vi "CG test stand Loadcell calibration.vi"() -> ()   [LabVIEW 2020]
doc: "This example demonstrates how to read N channels of analog input from a LINX device."
uses:
  <vilib>/MakerHub/LINX/Public/Peripherals/Analog/Analog Read N Chans.vi
  <vilib>/MakerHub/LINX/Private/Local IO/LinxAnalogRead.vi
  <vilib>/MakerHub/LINX/Public/Utilities/Check Channel.vi
  <vilib>/MakerHub/LINX/Public/Utilities/Open Serial.vi
  <vilib>/MakerHub/LINX/Private/Utilties/Generate Error.vi
  <vilib>/Analysis/Matrix/Numeric/Conversions/Array To Matrix - RA.vi
  <vilib>/Utility/file.llb/Write Delimited Spreadsheet (DBL).vi
  <vilib>/MakerHub/LINX/LMH-LINX.lvlib
  <vilib>/Analysis/Matrix/NI_Matrix.lvlib
panel:
  out "Unfiltered":dbl(graph)
  in  "Current Weight":dbl
  out "Filtered Data":dbl
  out "WRITING TO FILE":bool
  in  "?":bool
  out "error out":errorcluster
  out "Full filepath":string
  in  "Path":path
  in  "File extension":string
  in  "Filename":string
  in  "Analog Port":dbl
  out "Time Stamp":timestamp
  out "Filtered":dynamicdata(graph)
  out "Voltage":dbl
  in  "Stop Button":bool
  out "Loop Rate (Hz)":u32
  in  "Serial Port":refnum<visa-resource-name>
  # "X"
  # "+"
  # "CG test stand analog read\n\nThis VI works to read one single voltage value from an Arduino. Currently configured for a Mega 2560."
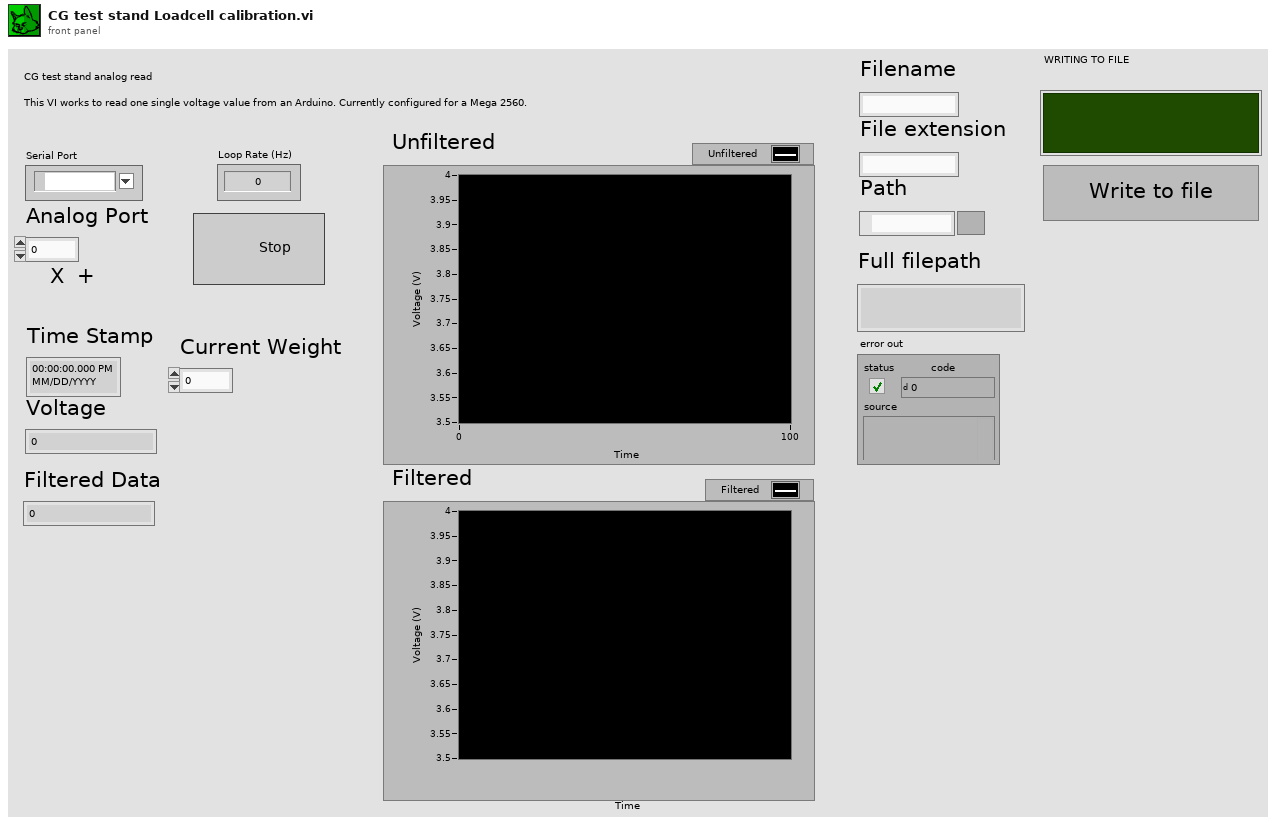
[diagram p1: front panel]
types:
  T1 = typedef "LMH-LINX.lvlib/LINX Ref.ctl" = cluster{"IO":T2, "Interface":T3, "LINX Device Config":T4}
  T2 = typedef "LMH-LINX.lvlib/Platform.ctl" = enum16{"Remote", "Local"}
  T3 = typedef "LMH-LINX.lvlib/Interface.ctl" = enum16{"Serial", "TCP"}
  T4 = typedef "LMH-LINX.lvlib/Device.lvlib/LINX Device Config.ctl" = cluster{"Interface":T3, "COM Port":refnum<visa-resource-name>, "TCP Configuration":T5, "Device Family":u8, "Device ID":u8, "Device Name":string, "TCP Ref":refnum<k5>, "Channels":T6}
  T5 = typedef "LMH-LINX.lvlib/Device.lvlib/TCP Config.ctl" = cluster{"IP Address":string, "Port":u16}
  T6 = typedef "LMH-LINX.lvlib/Channels.ctl" = cluster{"DI":u8[], "DO":u8[], "AI":u8[], "AO":u8[], "PWM":u8[], "QE":u8[], "UART":u8[], "I2C 2":u8[], "SPI":u8[], "CAN":u8[], "Servo":u8[], "AI Ref (V)":dbl, "AI Resolution (Bits)":u8, "AO Ref (V)":dbl, "AO Resolution (Bits)":u8}
  T7 = typedef "NI_Matrix.lvlib/RealMatrix.ctl" = dbl[][]
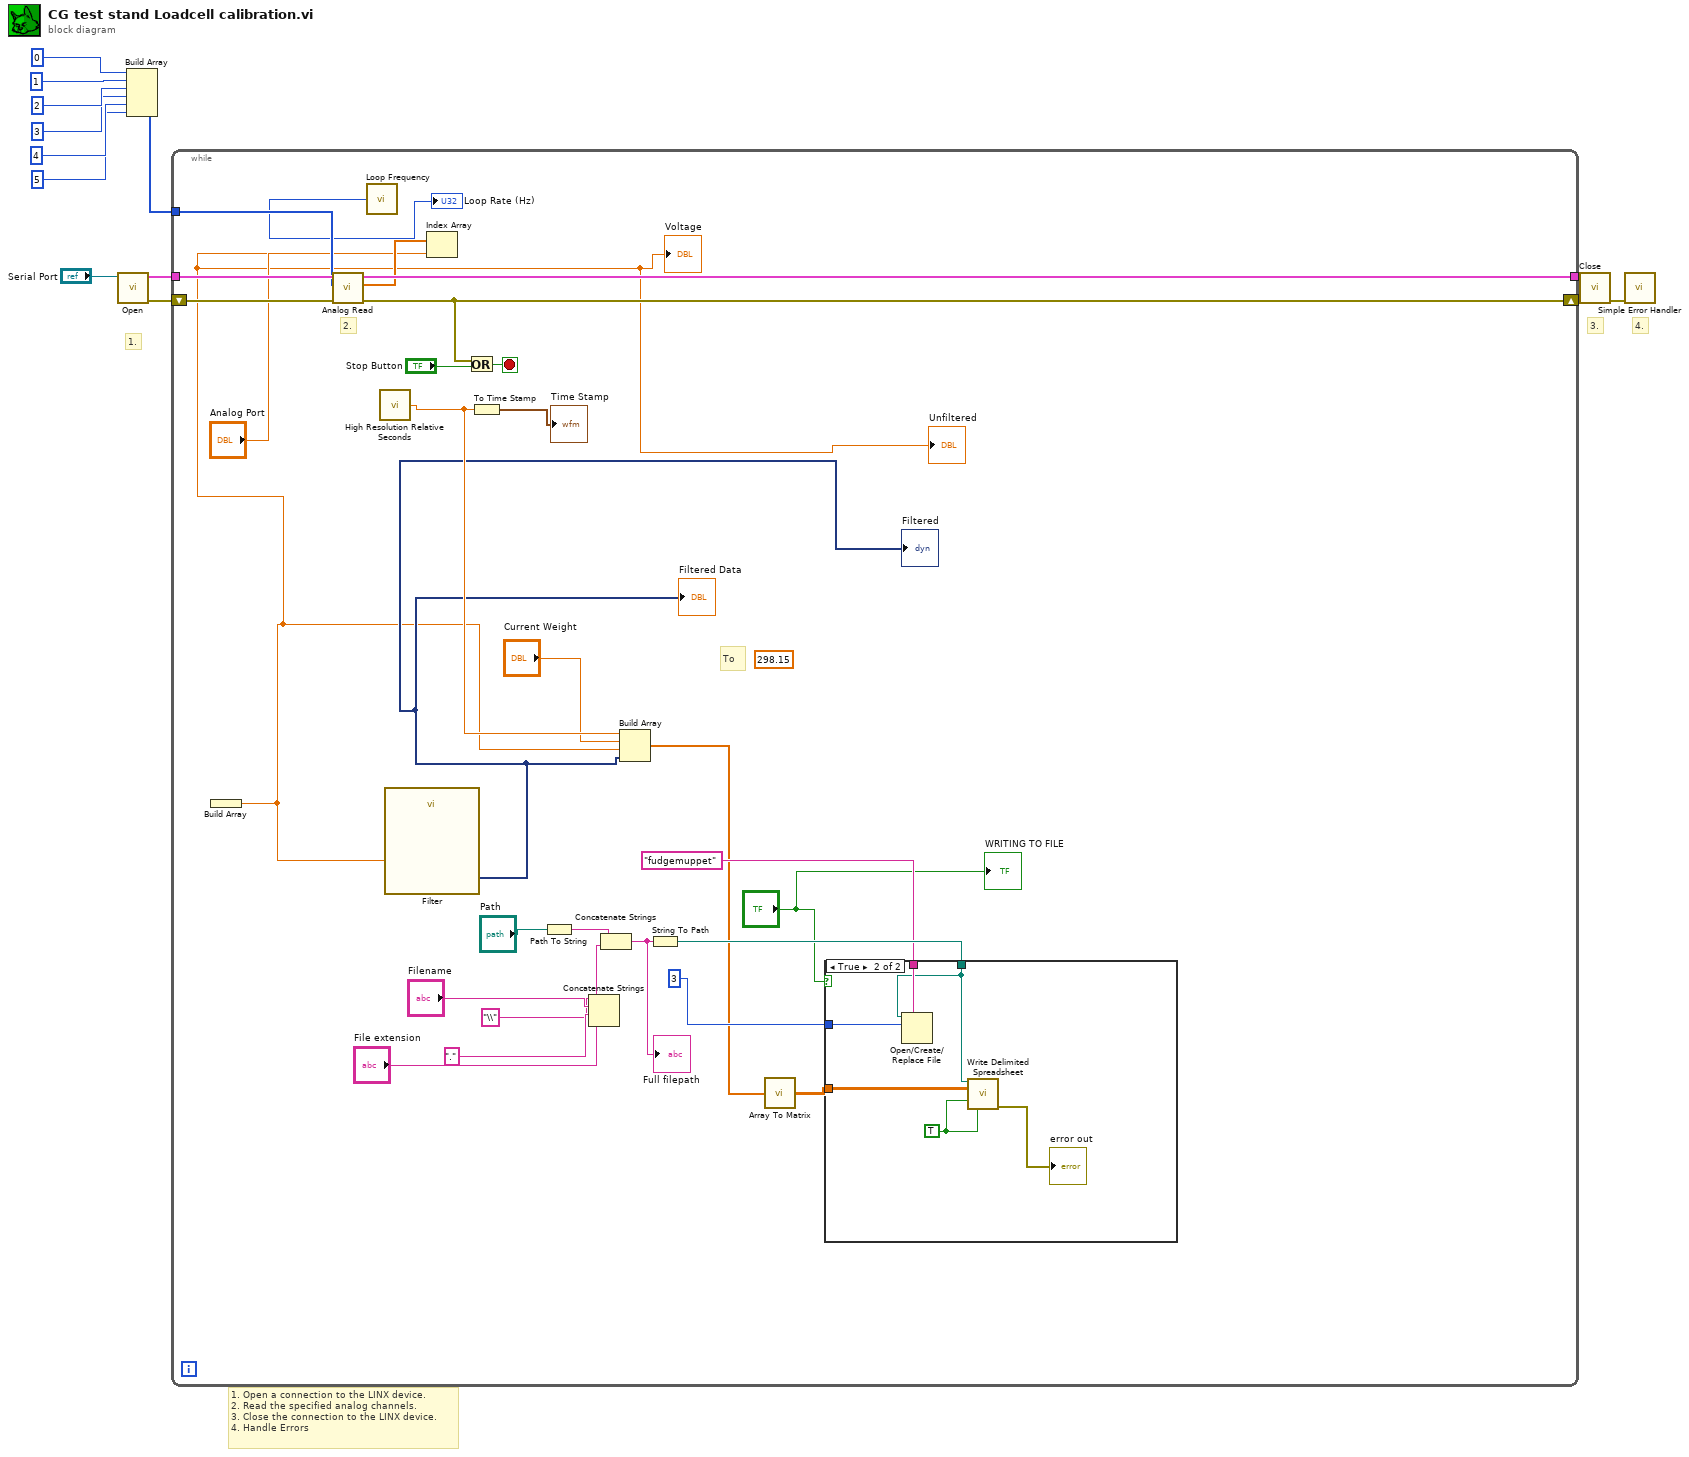
[diagram p0: block diagram]
diagram:
  # "1. Open a connection to the LINX device.\n2. Read the specified analog channels.\n3. Close the connection to the LINX device.\n4. Handle Errors"
  # "4."
  # "3."
  # "1."
  n1 = call-poly <vilib>:"Open.vi"("Serial Port"="Serial Port") -> ("Error Out"=w12:errorcluster, "LINX Resource"=w13:T1)  [unwired: 8 in, 1 out]
  n2 = Build Array(0, 1, 2, 3, 4, 5) -> (w7:i32[])
  n3 = while {
    tunnel: w13 -> [w42]
    tunnel: [w40] -> w11
    shift-right: [w37] -> w10
    shift-left: w12 -> [w41]
    tunnel: w7 -> [w36]
    stop <- w39 stop-if-true
    (unwired) 298.15
    # "To"
    # "2."
    n4 = call-poly <vilib>:"Analog Read.vi"("Error In"=w41, "AI Channel(s)"=w36, "LINX Resource"=w42) -> ("Error Out"=w37:errorcluster, "Voltages"=w35:dbl[], "LINX Resource"=w40:T1)  [unwired: 5 in, 1 out]
    n5 = call <vilib>:"Loop Frequency.vi"() -> ("Loop Rate (Hz)"=→"Loop Rate (Hz)":u32)
    n6 = call <vilib>:"High Resolution Relative Seconds.vi"() -> ("relative seconds"=w18:dbl)
    n7 = Index Array(array=w35, index="Analog Port") -> (element=w14:dbl)
    "Voltage" <- w14
    "Unfiltered" <- w14
    n8 = Build Array(w14) -> ()  [unwired: 1 out]
    n9 = call "Filter"("Signal"=w14) -> ("Filtered Signal"=w15:dynamicdata)  [unwired: 9 in, 1 out]
    "Filtered" <- w15
    "Filtered Data" <- w15
    n10 = Or(x=w37, y="Stop Button") -> (x .or. y?=w39:bool)
    n11 = To Time Stamp(1:w18) -> (0:→"Time Stamp":timestamp)
    n12 = Path To String(path="Path") -> (string=w31:string)
    n13 = Concatenate Strings("\\", "Filename", ".", "File extension") -> (w30:string)
    n14 = Concatenate Strings(w31, w30) -> (w29:string)
    "Full filepath" <- w29
    n15 = Build Array(w18, "Current Weight", w14, w15) -> (w19:dbl[])
    n16 = String To Path(string=w29) -> (path=w24:path)
    n17 = call-poly <vilib>:"Array To Matrix.vi"("Real 1D Array"=w19) -> ("Real Matrix (Column Vector)"=w20:T7)
    n18 = case shown="True" "?" {
      tunnel: w24 -> [_ w46]
      tunnel: w20 -> [_ w43]
      tunnel: "fudgemuppet" -> [_ w48]
      tunnel: 3 -> [_ w47]
      frame False {
      }
      frame True {
        w44 = TRUE
        n19 = Open/Create/Replace File(file path (use dialog)=w46, prompt=w48, operation (0:open)=w47) -> ()  [unwired: 3 in, 3 out]
        n20 = call-poly <vilib>:"Write Delimited Spreadsheet.vi"("file path (dialog if empty)"=w46, "2D data"=w43, "append to file? (new file:F)"=w44, "transpose? (no:F)"=w44) -> ("error out"=→"error out":errorcluster)  [unwired: 10 in, 1 out]
      }
    }
    "WRITING TO FILE" <- "?"
  }
  n21 = call <vilib>:"Close.vi"("Error In"=w10, "LINX Resource"=w11) -> ("Error Out"=w8:errorcluster)  [unwired: 9 in]
  n22 = call <vilib>:"Simple Error Handler.vi"("error in (no error)"=w8) -> ()  [unwired: 4 in, 5 out]
